vi "Autonomous Independent.vi"() -> ()   [LabVIEW 2017]
doc: "This VI is called when autonomous begins, and will automatically be terminated when autonomous ends. You can carry out timed or sensor driven robot movement independently without needing to return to the caller."
uses:
  Control 1.ctl
  Motion_Profiler_Class/Motion_Profiler_Class-323eb47bd4286328f3a3e236ed86bebf76c73fb1/MotionProfiles.lvclass
  <vilib>/Platform/TimedLoop/XDataNode/timing_clust.ctl
  <vilib>/Platform/TimedLoop/XDataNode/nitl_modes.ctl
  <vilib>/Platform/TimedLoop/XDataNode/wakeup.ctl
  <vilib>/Rock Robotics/WPI/Utilities/WPI_GetSetVariantRefNum.vi
  <vilib>/Rock Robotics/Network Tables/NT Write Numeric Array.vi
  <vilib>/Rock Robotics/Network Tables/NT Read String.vi
  UpperSwitchPressed.vi
  <vilib>/Platform/TimedLoop/XDataNode/XDataNode.xnode
  <vilib>/Platform/TimedLoop/XDataNode/XDNodeRunTimeDep.lvlib
panel:
  out "timer 2":u32=2247064
  out "AutoMode":string="LeftSwitch"
  out "MP Is Done Left":bool
  out "MP Is Done Right":bool
  in  "P_Right":dbl=0.25
  in  "I_Right":dbl
  in  "D_Right":dbl
  in  "F_Right":dbl=0.12
  in  "F_Left":dbl=0.12
  in  "D_Left":dbl
  in  "I_Left":dbl
  in  "P_Left":T1=0.19
  out "Right Bottom Buf Count":i32=5
  out "Right Is Under Run":bool
  out "Left Bottom Buf Count":i32=4
  out "Left Is Under Run":bool
  out "Left Vel":T2(graph)={"Set_Vel_(u/100ms)"=-8588, "Act_Vel_(u/100ms)"=-7311}
  out "Numeric":i32=26
  out "Right Vel":T2(graph)={"Set_Vel_(u/100ms)"=-8603, "Act_Vel_(u/100ms)"=-7623}
  out "Right Pos":T2(graph)={"Set_Vel_(u/100ms)"=-90788, "Act_Vel_(u/100ms)"=-97839}
  out "Left Pos":T2(graph)={"Set_Vel_(u/100ms)"=-72192, "Act_Vel_(u/100ms)"=-77390}
  out "Right Throttle":dbl(graph)=-0.9902248289345064
  out "Left Throttle":dbl(graph)=0.13880742913000976
  # "Be sure to right-click and choose Data Operations>>Make Current Value default if you want to save the array values with the VI"
  # "Left P gain: 0.21, Right P Gain 0.25 -> before 09/12/18\nLeft Gain :0.205, Right Gain .25 - > 09/12/18 -> Tuned after changing center drop for center grove practice"
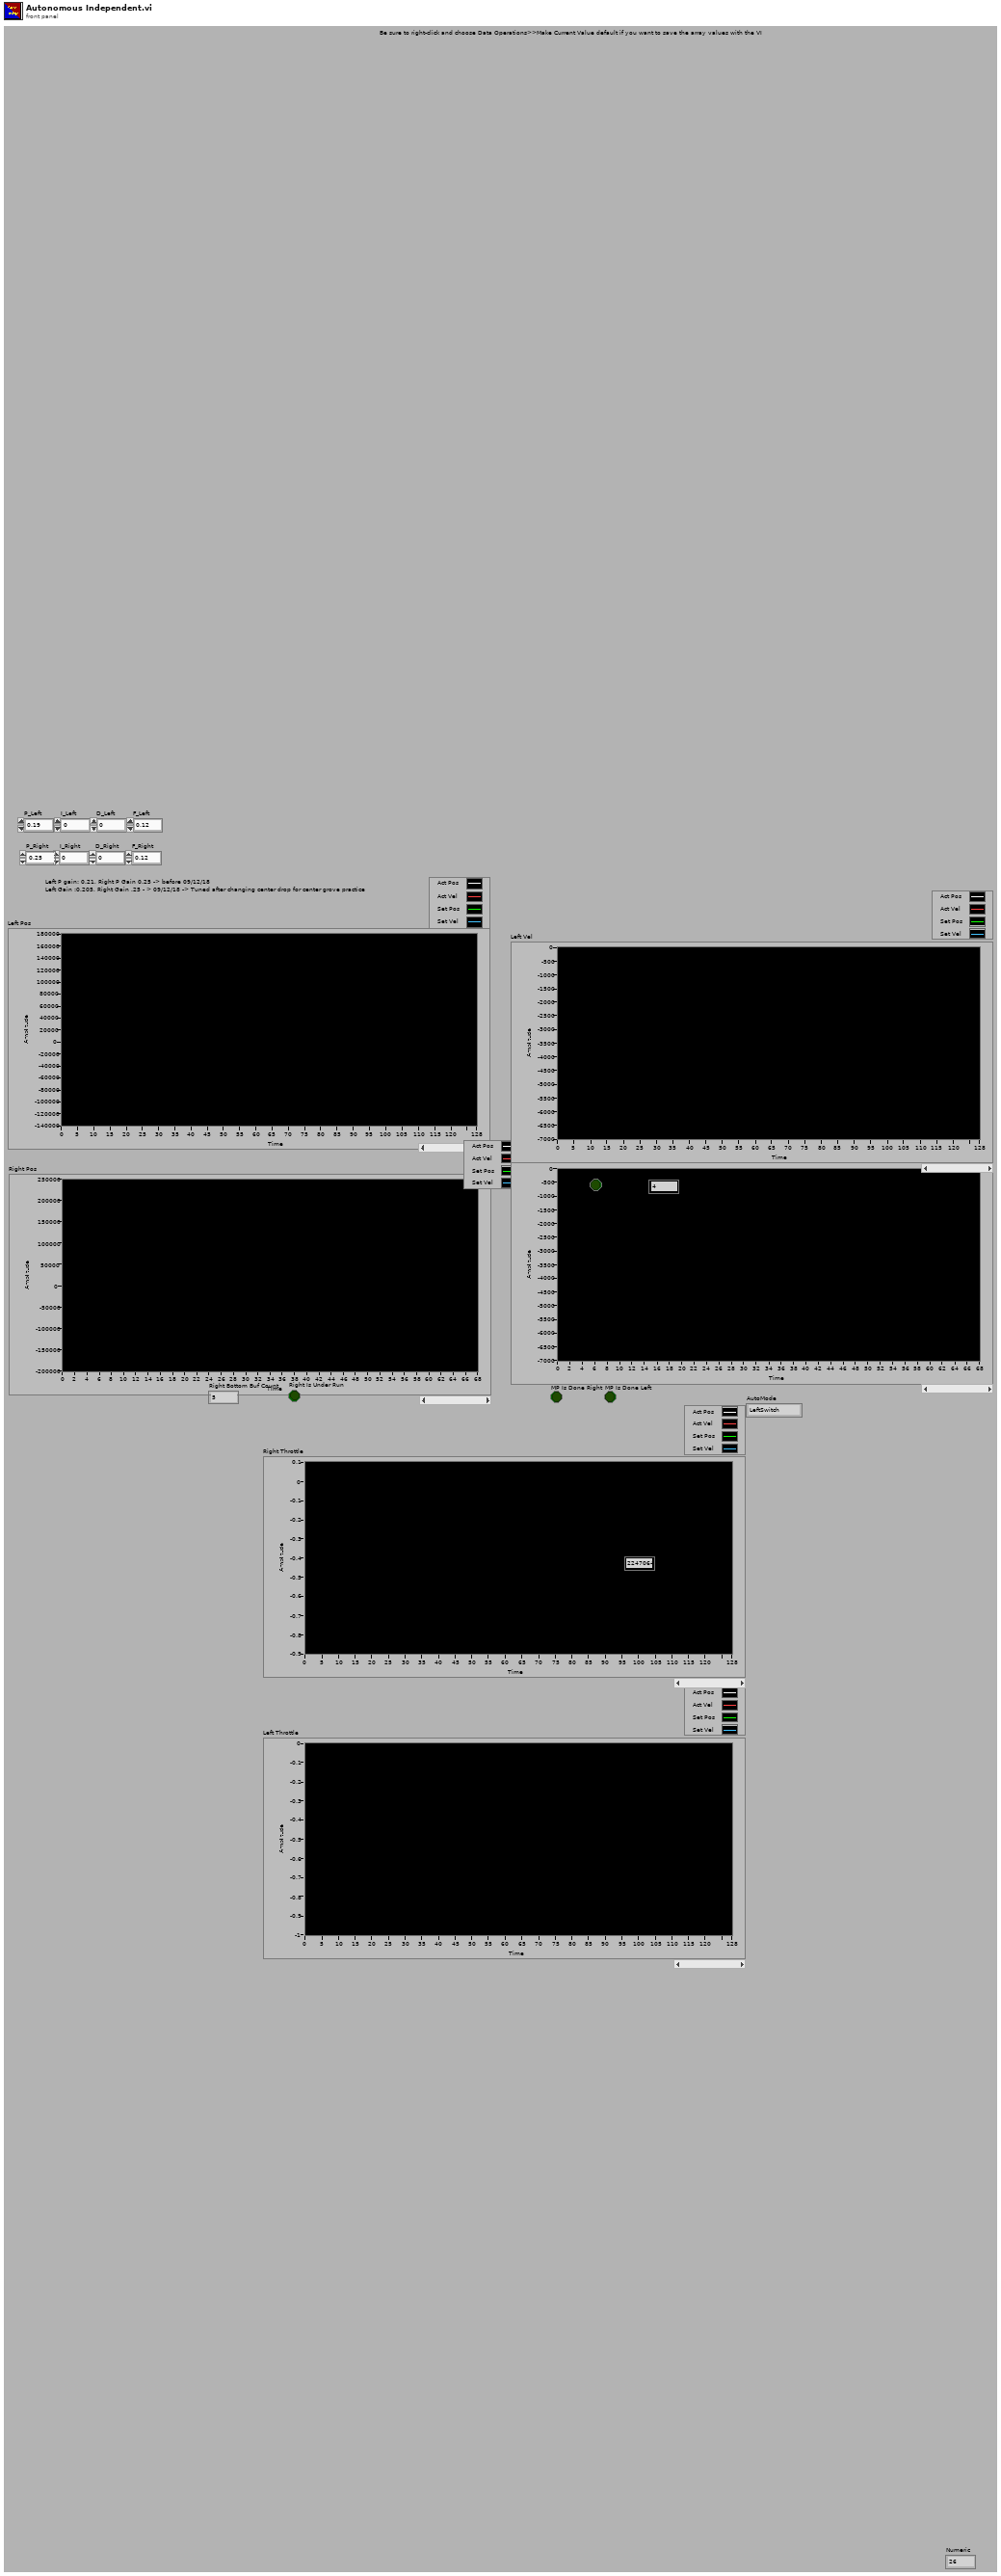
[diagram p1: front panel]
types:
  T1 = typedef "Control 1.ctl" = dbl
  T2 = cluster{"Set_Vel_(u/100ms)":i32, "Act_Vel_(u/100ms)":i32}
  T3 = typedef "WPI_JoystickDevRef.ctl" = cluster{"Device":T4}
  T4 = typedef "WPI_JoystickDeviceEnum.ctl" = enum16{"USB 0", "USB 1", "USB 2", "USB 3", "USB 4", "USB 5"}
  T5 = typedef "WPI_MotorControlDeviceRef.ctl" = cluster{"DeviceStatus":errorcluster, "Type":T6, "PWM":cluster{"PWM Channel":T7, "DeadBand":T8}, "CAN":cluster{"Device Number":u8, "SetOutput VI Ref":variant, "GetOutput VI Ref":variant, "Enable VI Ref":variant, "Disable VI Ref":variant, "Data":variant}, "Invert":bool, "DIO PWM":cluster{"PWM \"Enable\" Channel":T7, "DIOChannel":T9, "PWM Rate":dbl}}
  T6 = typedef "WPI_MotorControlType.ctl" = enum16{"PWM", "CAN", "DIO PWM"}
  T7 = typedef "FPGA_DIOPWMChannel.ctl" = enum8{"PWM 0", "PWM 1", "PWM 2", "PWM 3", "PWM 4", "PWM 5", "PWM 6", "PWM 7", "PWM 8", "PWM 9", "PWM MXP 0", "PWM MXP 1", "PWM MXP 2", "PWM MXP 3", "PWM MXP 4", "PWM MXP 5", "PWM MXP 6", "PWM MXP 7", "PWM MXP 8", "PWM MXP 9", "Invalid"}
  T8 = typedef "WPI_PWMDeadband.ctl" = cluster{"Name":string, "maxPositivePwm":i32, "minPositivePwm":i32, "centerPwm":i32, "maxNegativePwm":i32, "minNegativePwm":i32, "angularRange":u16}
  T9 = typedef "FPGA_DIOChannel.ctl" = enum8{"DIO 0", "DIO 1", "DIO 2", "DIO 3", "DIO 4", "DIO 5", "DIO 6", "DIO 7", "DIO 8", "DIO 9", "DIO MXP 0", "DIO MXP 1", "DIO MXP 2", "DIO MXP 3", "DIO MXP 4", "DIO MXP 5", "DIO MXP 6", "DIO MXP 7", "DIO MXP 8", "DIO MXP 9", "DIO MXP 10", "DIO MXP 11", "DIO MXP 12", "DIO MXP 13", "DIO MXP 14", "DIO MXP 15", "SPI Port CS1", "SPI Port CS2", "SPI Port CS3", "SPI Port MISO", "SPI Port MOSI", "Invalid"}
  T10 = typedef "XDNodeRunTimeDep.lvlib/timing_clust.ctl" = cluster{"Expected End [f-1]":u64, "Actual End [f-1]":u64, "Finished Late? [f-1]":bool, "Expected End [i-1]":u64, "Actual End [i-1]":u64, "Finished Late? [i-1]":bool, "Expected Start [i]":u64, "Actual Start [i]":u64, "Expected Start [f]":u64, "Actual Start [f]":u64, "Source Name":string, "Structure Name":string, "Period":i64, "Deadline":i64, "Offset":i64, "Start":i64, "Priority":i32, "Timeout":i32, "Mode":T11, "Wakeup Reason":T12, "Error":errorcluster, "Source Type":string, "Secondary Source Type":string, "Global End Time":u64, "Global Start Time":u64, "Frame Duration":u64, "Iteration Duration":u64, "Assigned CPU":i32, "I/O Scan Engine Mode":u32}
  T11 = typedef "XDNodeRunTimeDep.lvlib/nitl_modes.ctl" = enum32{"No Change", "Process missed periods, maintain original phase", "Discard missed periods, maintain original phase", "Process missed periods, ignore original phase", "Discard missed periods, ignore original phase"}
  T12 = typedef "XDNodeRunTimeDep.lvlib/wakeup.ctl" = enum32{"Normal", "Aborted", "Asynchronous wakeup", "Timing source error", "Timed loop error", "Timeout"}
  T13 = typedef "MotionProfiles.lvclass/MotionProfile_MP_Class_Status.ctl" = cluster{"Motion Profile Status":cluster{"Top Buffer Remaining":i32, "Top Buffer Count":i32, "Bottom Buffer Count":i32, "Has Underrun?":bool, "Is Underrun?":bool, "Active Point Valid?":bool, "Is Last?":bool, "Profile Slot Select 0":i32, "Output Enable":i32, "Time Duration (ms)":i32, "Profile Slot Select 1":i32}, "TalonState":T14, "MP Is Done":bool, "MP Is Executing":bool, "Set_Vel_(u/100ms)":i32, "Set_Pos_(u)":i32, "Act_Vel_(u/100ms)":i32, "Act_Pos(u)":i32, "Throtle":dbl}
  T14 = typedef "MotionProfiles.lvclass/MotionProfile_TalonSetValueEnum.ctl" = enum16{"Disable", "Enable", "Hold"}
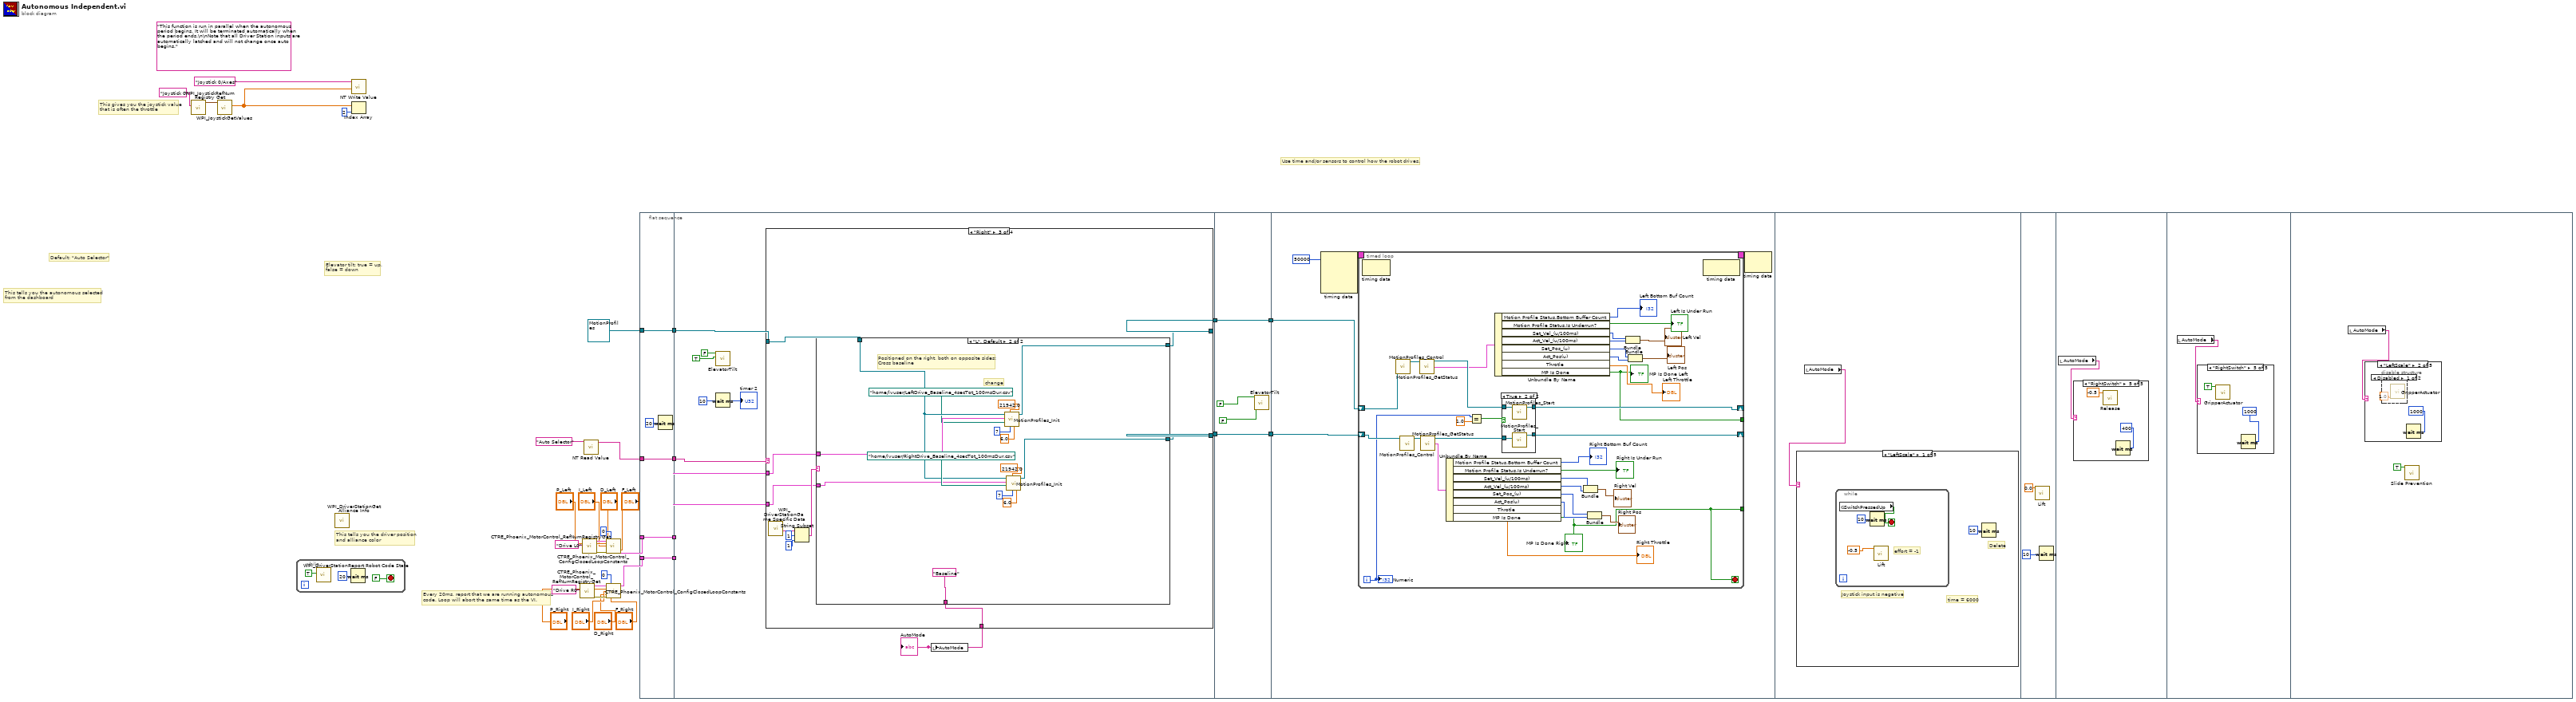
[diagram p0: block diagram]
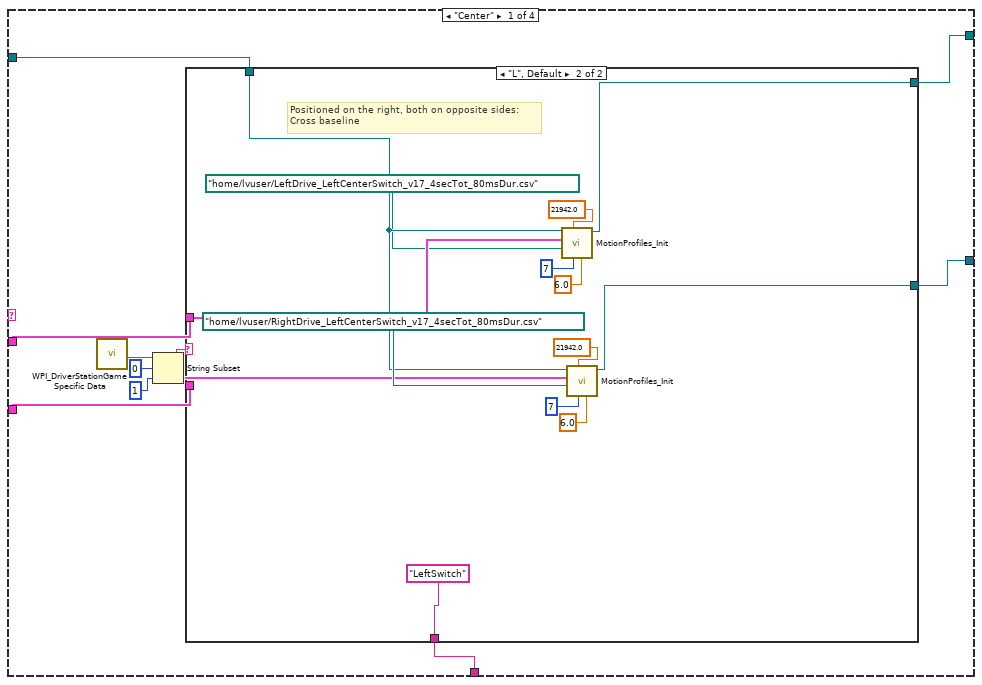
[diagram p2: hidden frame]
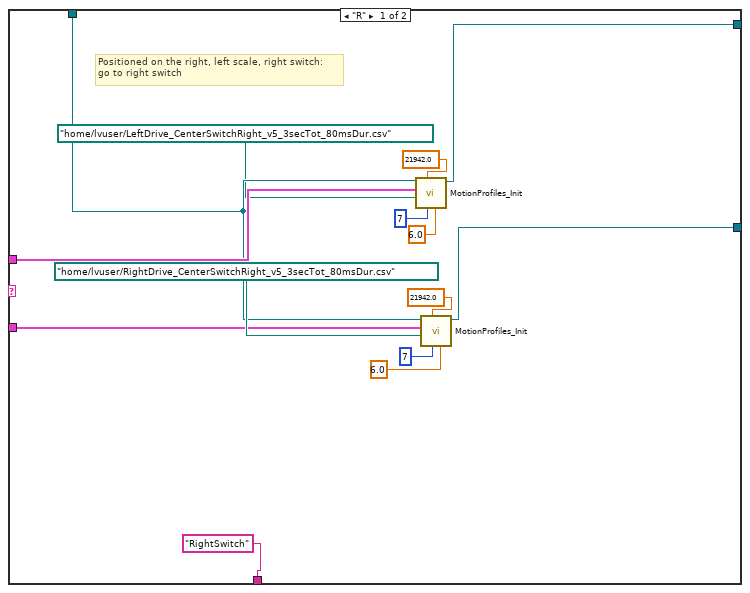
[diagram p3: hidden frame]
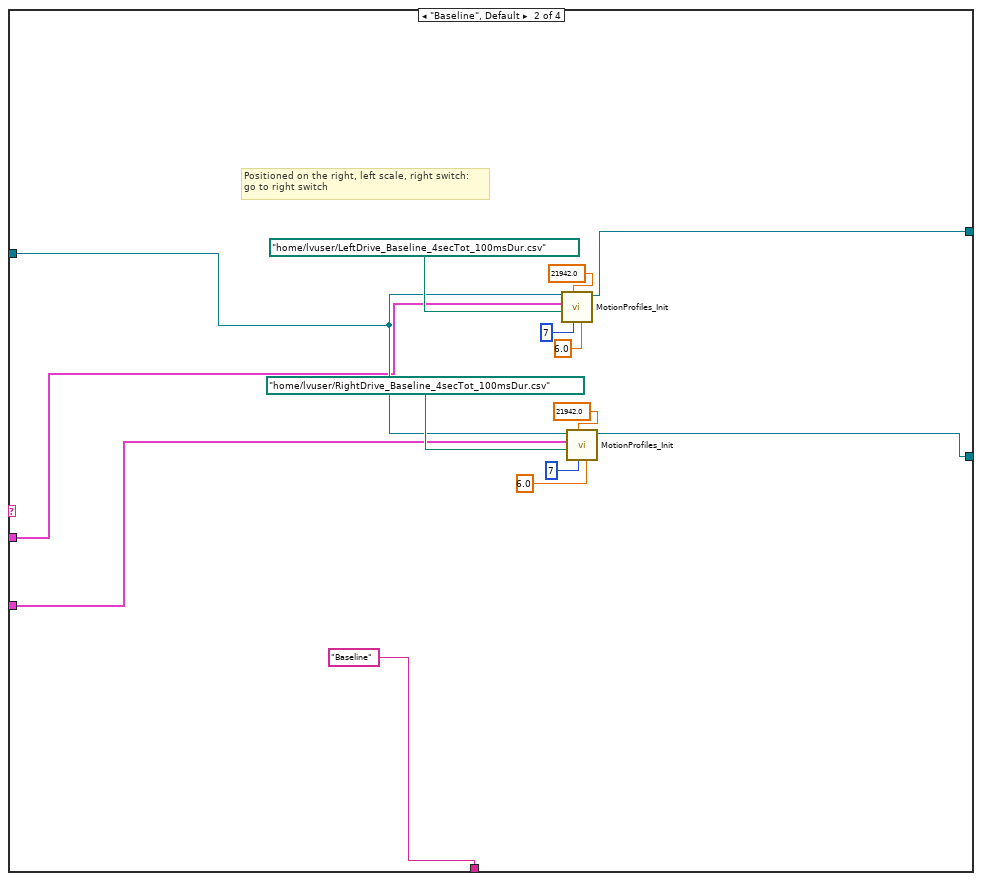
[diagram p4: hidden frame]
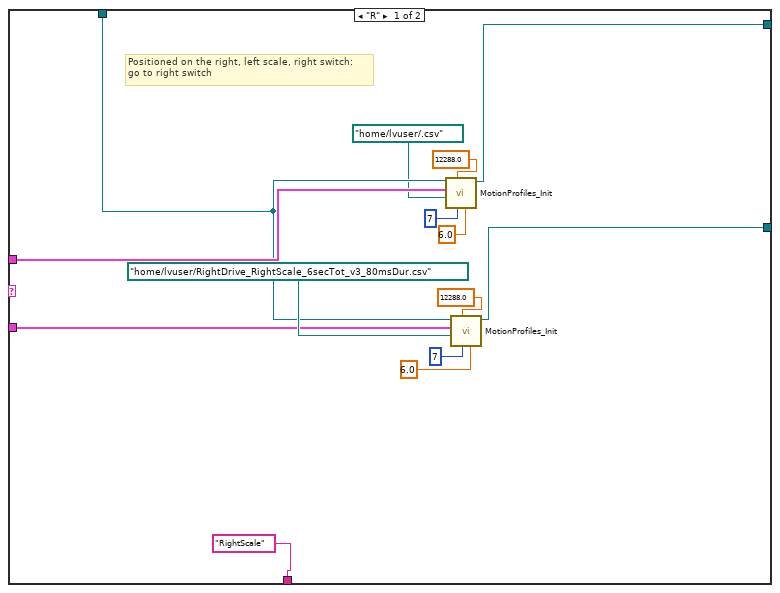
[diagram p5: hidden frame]
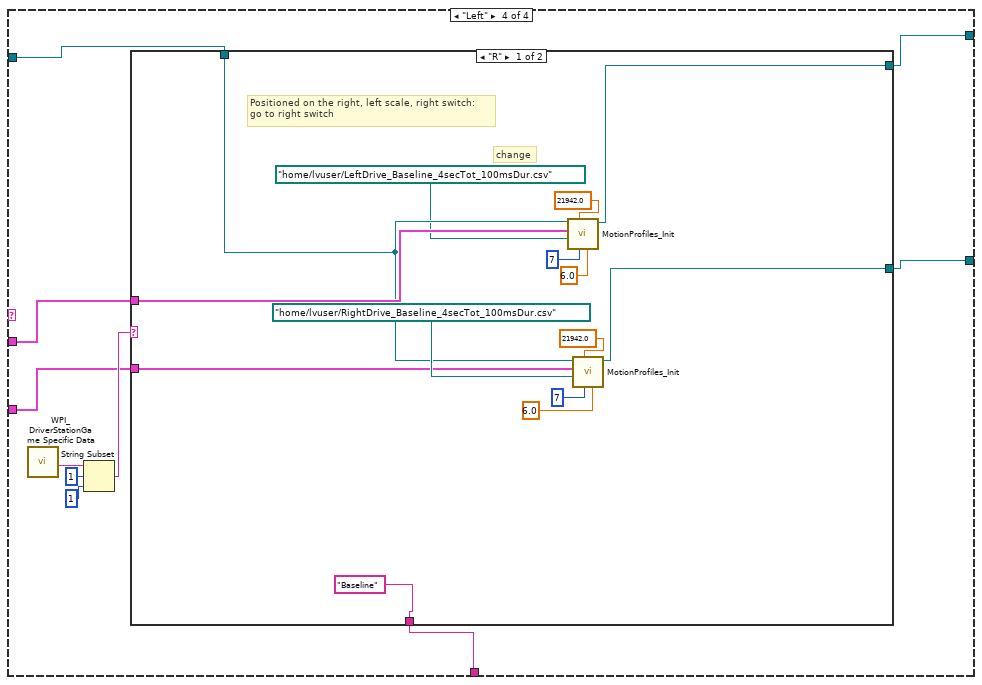
[diagram p6: hidden frame]
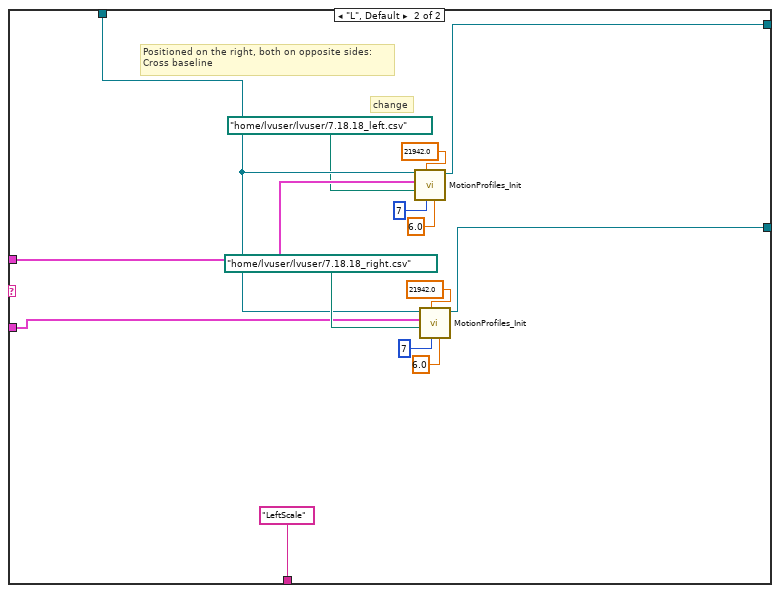
[diagram p7: hidden frame]
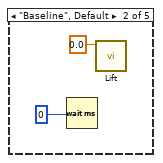
[diagram p9: hidden frame]
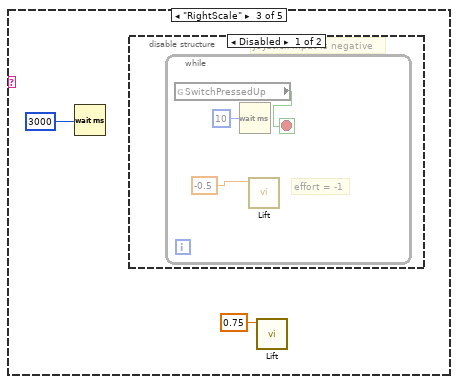
[diagram p10: hidden frame]
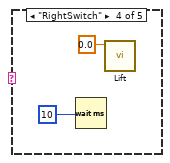
[diagram p12: hidden frame]
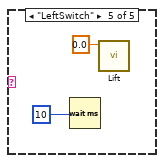
[diagram p13: hidden frame]
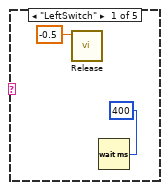
[diagram p14: hidden frame]
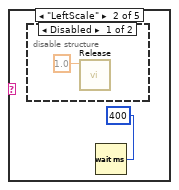
[diagram p15: hidden frame]
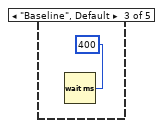
[diagram p17: hidden frame]
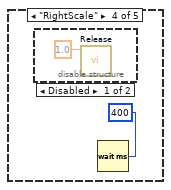
[diagram p18: hidden frame]
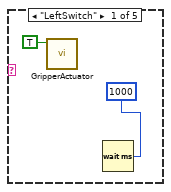
[diagram p20: hidden frame]
diagram:
  (unwired) "This function is run in parallel when the autonomous period begins. It will be terminated automatically when the period ends.\n\nNote that all Driver Station inputs are automatically latched and will not change once auto begins."
  # "Elevator tilt: true = up,\nfalse = down"
  # "Every 20ms, report that we are running autonomous\ncode. Loop will abort the same time as the VI."
  # "Default: \"Auto Selector\""
  # "This tells you the autonomous selected\nfrom the dashboard"
  # "This gives you the joystick value\nthat is often the throttle"
  # "Use time and/or sensors to control how the robot drives."
  # "This tells you the driver position\nand alliance color"
  n1 = call <vilib>:"WPI_JoystickRefNum Registry Get.vi"("refnum name"="Joystick 0") -> ("JoystickDevRef"=w33:T3)  [unwired: 1 in, 9 out]
  n2 = call <vilib>:"WPI_JoystickGetValues.vi"("JoystickDevRef"=w33) -> ("Axes"=w31:dbl[])  [unwired: 6 in, 4 out]
  n3 = while {
    stop <- FALSE stop-if-true
    n4 = call <vilib>:"WPI_DriverStationReport Robot Code State.vi"("Autonomous"=TRUE) -> ()  [unwired: 10 in, 1 out]
    n5 = Wait (ms)(milliseconds to wait=u32 20) -> ()  [unwired: 1 out]
  }
  n6 = call <vilib>:"WPI_DriverStationGet Alliance Info.vi"() -> ()  [unwired: 12 out]
  n7 = call-poly <vilib>:"NT Write Value.vi"("Numeric Array"=w31, "Name"="Joystick 0/Axes") -> ()  [unwired: 9 in, 1 out]
  n8 = Index Array(array=w31, index=2) -> ()  [unwired: 1 out]
  n9 = call <vilib>:"CTRE_Phoenix_MotorControl_RefNumRegistryGet.vi"("refnum name"="Drive R0") -> ("error out"=w21:errorcluster, "PhoenixMotorControlDevRef"=w22:T5)  [unwired: 9 in]
  n10 = call <vilib>:"CTRE_Phoenix_MotorControl_RefNumRegistryGet.vi"("refnum name"="Drive L0") -> ("error out"=w24:errorcluster, "PhoenixMotorControlDevRef"=w25:T5)  [unwired: 9 in]
  n11 = call-poly <vilib>:"NT Read Value.vi"("Name"="Auto Selector") -> ("String"=w5:string)  [unwired: 9 in, 1 out]
  n12 = call <vilib>:"CTRE_Phoenix_MotorControl_ConfigClosedLoopConstants.vi"("PhoenixMotorControlDevRef"=w25, "slotIdx"=0, "P"="P_Left", "I"="I_Left", "D"="D_Left", "error in (no error)"=w24, "F"="F_Left") -> ("PhoenixMotorControlDevRef"=w18:T5)  [unwired: 7 in, 1 out]
  n13 = call <vilib>:"CTRE_Phoenix_MotorControl_ConfigClosedLoopConstants.vi"("PhoenixMotorControlDevRef"=w22, "slotIdx"=0, "P"="P_Right", "I"="I_Right", "D"="D_Right", "error in (no error)"=w21, "F"="F_Right") -> ("PhoenixMotorControlDevRef"=w17:T5)  [unwired: 7 in, 1 out]
  n14 = flat-sequence {
    tunnel: w5 -> [w39]
    tunnel: refnum<class "MotionProfiles.lvclass"> refnum ("MotionProfiles.lvclass") -> [w40]
    tunnel: w17 -> [w41]
    tunnel: w18 -> [w42]
    tunnel: [w42] -> w10
    tunnel: [w41] -> w9
    tunnel: [w40] -> w8
    tunnel: [w39] -> w7
    tunnel: [w50] -> w2
    tunnel: [w51] -> w1
    tunnel: w10 -> [w53]
    tunnel: w9 -> [w52]
    tunnel: w8 -> [w49]
    tunnel: w7 -> [w47]
    tunnel: w2 -> [w185]
    tunnel: [w185] -> w4
    tunnel: w1 -> [w184]
    tunnel: [w184] -> w3
    tunnel: w4 -> [w190]
    tunnel: w3 -> [w189]
    frame #0 {
      n15 = Wait (ms)(milliseconds to wait=u32 20) -> ()  [unwired: 1 out]
    }
    frame #1 {
      n16 = call "ElevatorTilt.vi"("Down?"=TRUE, "Up"=FALSE) -> ()  [unwired: 10 in]
      n17 = Wait (ms)(milliseconds to wait=u32 10) -> (millisecond timer value=→"timer 2":u32)
      n18 = case shown="\"Right\"" w47 {
        tunnel: w53 -> [w62 w94 w110 w148]
        tunnel: w52 -> [w61 w93 w109 w147]
        tunnel: [w60 w95 w106 w144] -> w51
        tunnel: [w59 w96 w107 w145] -> w50
        tunnel: w49 -> [w55 w97 w115 w149]
        tunnel: [w54 "Baseline" w108 w146] -> w48
        frame "Center" {
          n19 = call <vilib>:"WPI_DriverStationGame Specific Data.vi"() -> ("Game Specific Data"=w63:string)  [unwired: 11 in]
          n20 = String Subset(string=w63, offset (0)=0, length (rest)=1 ("length (rest)")) -> (substring=w58:string)
          n21 = case shown="\"L\", Default" w58 {
            tunnel: w62 -> [w70 w83]
            tunnel: w61 -> [w69 w84]
            tunnel: [w68 w82] -> w59
            tunnel: [w67 w81] -> w60
            tunnel: w55 -> [w66 w80]
            tunnel: ["RightSwitch" "LeftSwitch"] -> w54
            frame "R" {
              # "Positioned on the right, left scale, right switch:\ngo to right switch"
              n22 = call "MotionProfiles_Init.vi"("Wheel_Diameter (in)"=6.0, "MP_Frame_Rate_(ms)"=7, "Encoder_CPR_4x"=21942.0, "CSV File Path"=path "/home/lvuser/LeftDrive_CenterSwitchRight_v5_3secTot_80msDur.csv", "PhoenixMotorControlDevRef"=w70, "MotionProfiles in"=w66) -> ("MotionProfiles out"=w68:refnum<class "MotionProfiles.lvclass">)  [unwired: 4 in, 1 out]
              n23 = call "MotionProfiles_Init.vi"("Wheel_Diameter (in)"=6.0, "MP_Frame_Rate_(ms)"=7, "Encoder_CPR_4x"=21942.0, "CSV File Path"=path "/home/lvuser/RightDrive_CenterSwitchRight_v5_3secTot_80msDur.csv", "PhoenixMotorControlDevRef"=w69, "MotionProfiles in"=w66) -> ("MotionProfiles out"=w67:refnum<class "MotionProfiles.lvclass">)  [unwired: 4 in, 1 out]
            }
            frame "L", Default {
              # "Positioned on the right, both on opposite sides:\nCross baseline"
              n24 = call "MotionProfiles_Init.vi"("Wheel_Diameter (in)"=6.0, "MP_Frame_Rate_(ms)"=7, "Encoder_CPR_4x"=21942.0, "CSV File Path"=path "/home/lvuser/LeftDrive_LeftCenterSwitch_v17_4secTot_80msDur.csv", "PhoenixMotorControlDevRef"=w83, "MotionProfiles in"=w80) -> ("MotionProfiles out"=w82:refnum<class "MotionProfiles.lvclass">)  [unwired: 4 in, 1 out]
              n25 = call "MotionProfiles_Init.vi"("Wheel_Diameter (in)"=6.0, "MP_Frame_Rate_(ms)"=7, "Encoder_CPR_4x"=21942.0, "CSV File Path"=path "/home/lvuser/RightDrive_LeftCenterSwitch_v17_4secTot_80msDur.csv", "PhoenixMotorControlDevRef"=w84, "MotionProfiles in"=w80) -> ("MotionProfiles out"=w81:refnum<class "MotionProfiles.lvclass">)  [unwired: 4 in, 1 out]
            }
          }
        }
        frame "Baseline", Default {
          # "Positioned on the right, left scale, right switch:\ngo to right switch"
          n26 = call "MotionProfiles_Init.vi"("Wheel_Diameter (in)"=6.0, "MP_Frame_Rate_(ms)"=7, "Encoder_CPR_4x"=21942.0, "CSV File Path"=path "/home/lvuser/LeftDrive_Baseline_4secTot_100msDur.csv", "PhoenixMotorControlDevRef"=w94, "MotionProfiles in"=w97) -> ("MotionProfiles out"=w96:refnum<class "MotionProfiles.lvclass">)  [unwired: 4 in, 1 out]
          n27 = call "MotionProfiles_Init.vi"("Wheel_Diameter (in)"=6.0, "MP_Frame_Rate_(ms)"=7, "Encoder_CPR_4x"=21942.0, "CSV File Path"=path "/home/lvuser/RightDrive_Baseline_4secTot_100msDur.csv", "PhoenixMotorControlDevRef"=w93, "MotionProfiles in"=w97) -> ("MotionProfiles out"=w95:refnum<class "MotionProfiles.lvclass">)  [unwired: 4 in, 1 out]
        }
        frame "Right" {
          n28 = call <vilib>:"WPI_DriverStationGame Specific Data.vi"() -> ("Game Specific Data"=w114:string)  [unwired: 11 in]
          n29 = String Subset(string=w114, offset (0)=1, length (rest)=1 ("length (rest)")) -> (substring=w111:string)
          n30 = case shown="\"L\", Default" w111 {
            tunnel: w110 -> [w122 w135]
            tunnel: w109 -> [w121 w136]
            tunnel: [w120 w134] -> w107
            tunnel: [w119 w133] -> w106
            tunnel: w115 -> [w118 w132]
            tunnel: ["RightScale" "Baseline"] -> w108
            frame "R" {
              # "Positioned on the right, left scale, right switch:\ngo to right switch"
              n31 = call "MotionProfiles_Init.vi"("Wheel_Diameter (in)"=6.0, "MP_Frame_Rate_(ms)"=7, "Encoder_CPR_4x"=12288.0, "CSV File Path"=path "/home/lvuser/.csv", "PhoenixMotorControlDevRef"=w122, "MotionProfiles in"=w118) -> ("MotionProfiles out"=w120:refnum<class "MotionProfiles.lvclass">)  [unwired: 4 in, 1 out]
              n32 = call "MotionProfiles_Init.vi"("Wheel_Diameter (in)"=6.0, "MP_Frame_Rate_(ms)"=7, "Encoder_CPR_4x"=12288.0, "CSV File Path"=path "/home/lvuser/RightDrive_RightScale_6secTot_v3_80msDur.csv", "PhoenixMotorControlDevRef"=w121, "MotionProfiles in"=w118) -> ("MotionProfiles out"=w119:refnum<class "MotionProfiles.lvclass">)  [unwired: 4 in, 1 out]
            }
            frame "L", Default {
              # "change"
              # "Positioned on the right, both on opposite sides:\nCross baseline"
              n33 = call "MotionProfiles_Init.vi"("Wheel_Diameter (in)"=6.0, "MP_Frame_Rate_(ms)"=7, "Encoder_CPR_4x"=21942.0, "CSV File Path"=path "/home/lvuser/LeftDrive_Baseline_4secTot_100msDur.csv", "PhoenixMotorControlDevRef"=w135, "MotionProfiles in"=w132) -> ("MotionProfiles out"=w134:refnum<class "MotionProfiles.lvclass">)  [unwired: 4 in, 1 out]
              n34 = call "MotionProfiles_Init.vi"("Wheel_Diameter (in)"=6.0, "MP_Frame_Rate_(ms)"=7, "Encoder_CPR_4x"=21942.0, "CSV File Path"=path "/home/lvuser/RightDrive_Baseline_4secTot_100msDur.csv", "PhoenixMotorControlDevRef"=w136, "MotionProfiles in"=w132) -> ("MotionProfiles out"=w133:refnum<class "MotionProfiles.lvclass">)  [unwired: 4 in, 1 out]
            }
          }
        }
        frame "Left" {
          n35 = call <vilib>:"WPI_DriverStationGame Specific Data.vi"() -> ("Game Specific Data"=w153:string)  [unwired: 11 in]
          n36 = String Subset(string=w153, offset (0)=1, length (rest)=1 ("length (rest)")) -> (substring=w150:string)
          n37 = case shown="\"R\"" w150 {
            tunnel: w148 -> [w160 w173]
            tunnel: w147 -> [w159 w174]
            tunnel: [w158 w172] -> w145
            tunnel: [w157 w171] -> w144
            tunnel: w149 -> [w156 w170]
            tunnel: ["Baseline" "LeftScale"] -> w146
            frame "R" {
              # "change"
              # "Positioned on the right, left scale, right switch:\ngo to right switch"
              n38 = call "MotionProfiles_Init.vi"("Wheel_Diameter (in)"=6.0, "MP_Frame_Rate_(ms)"=7, "Encoder_CPR_4x"=21942.0, "CSV File Path"=path "/home/lvuser/LeftDrive_Baseline_4secTot_100msDur.csv", "PhoenixMotorControlDevRef"=w160, "MotionProfiles in"=w156) -> ("MotionProfiles out"=w158:refnum<class "MotionProfiles.lvclass">)  [unwired: 4 in, 1 out]
              n39 = call "MotionProfiles_Init.vi"("Wheel_Diameter (in)"=6.0, "MP_Frame_Rate_(ms)"=7, "Encoder_CPR_4x"=21942.0, "CSV File Path"=path "/home/lvuser/RightDrive_Baseline_4secTot_100msDur.csv", "PhoenixMotorControlDevRef"=w159, "MotionProfiles in"=w156) -> ("MotionProfiles out"=w157:refnum<class "MotionProfiles.lvclass">)  [unwired: 4 in, 1 out]
            }
            frame "L", Default {
              # "change"
              # "Positioned on the right, both on opposite sides:\nCross baseline"
              n40 = call "MotionProfiles_Init.vi"("Wheel_Diameter (in)"=6.0, "MP_Frame_Rate_(ms)"=7, "Encoder_CPR_4x"=21942.0, "CSV File Path"=path "/home/lvuser/lvuser/7.18.18_left.csv", "PhoenixMotorControlDevRef"=w173, "MotionProfiles in"=w170) -> ("MotionProfiles out"=w172:refnum<class "MotionProfiles.lvclass">)  [unwired: 4 in, 1 out]
              n41 = call "MotionProfiles_Init.vi"("Wheel_Diameter (in)"=6.0, "MP_Frame_Rate_(ms)"=7, "Encoder_CPR_4x"=21942.0, "CSV File Path"=path "/home/lvuser/lvuser/7.18.18_right.csv", "PhoenixMotorControlDevRef"=w174, "MotionProfiles in"=w170) -> ("MotionProfiles out"=w171:refnum<class "MotionProfiles.lvclass">)  [unwired: 4 in, 1 out]
            }
          }
        }
      }
      "AutoMode" <- w48
      n42 = local write "AutoMode"(w48) -> ()
    }
    frame #2 {
      n43 = call "ElevatorTilt.vi"("Down?"=FALSE, "Up"=FALSE) -> ()  [unwired: 10 in]
    }
    frame #3 {
      n44 = node-c288(50000) -> (w188:T10)  [unwired: 3 in]
      n45 = timed-loop {
        timing: w188 -> [_]
        timing-out: [_] -> w187
        shift-right: [w211] -> _
        shift-left: w189 -> [w209]
        shift-right: [w210] -> _
        shift-left: w190 -> [w193]
        tunnel: [w191] -> _
        tunnel: [w192] -> _
        i -> [w206]
        stop <- w191 stop-if-true
        n46 = node-c288() -> ()  [unwired: 1 in, 1 out]
        n47 = call "MotionProfiles_Control.vi"("MotionProfiles in"=w193) -> ("MotionProfiles out"=w223:refnum<class "MotionProfiles.lvclass">)  [unwired: 9 in, 1 out]
        n48 = call "MotionProfiles_Control.vi"("MotionProfiles in"=w209) -> ("MotionProfiles out"=w222:refnum<class "MotionProfiles.lvclass">)  [unwired: 9 in, 1 out]
        n49 = call "MotionProfiles_GetStatus.vi"("MotionProfiles in"=w223) -> ("MotionProfiles out"=w220:refnum<class "MotionProfiles.lvclass">, "MP_Class_Status"=w218:T13)  [unwired: 12 in, 1 out]
        n50 = call "MotionProfiles_GetStatus.vi"("MotionProfiles in"=w222) -> ("MotionProfiles out"=w221:refnum<class "MotionProfiles.lvclass">, "MP_Class_Status"=w219:T13)  [unwired: 12 in, 1 out]
        n51 = Unbundle By Name(w219) -> ("Motion Profile Status.Bottom Buffer Count"=→"Right Bottom Buf Count":i32, "Motion Profile Status.Is Underrun?"=→"Right Is Under Run":bool, "Set_Vel_(u/100ms)"=w203:i32, "Act_Vel_(u/100ms)"=w202:i32, "Set_Pos_(u)"=w200:i32, "Act_Pos(u)"=w199:i32, "Throtle"=→"Right Throttle":dbl, "MP Is Done"=w191:bool)
        "MP Is Done Right" <- w191
        n52 = Equal?(x=w206, y=1.0) -> (x = y?=w208:bool)
        n53 = Unbundle By Name(w218) -> ("Motion Profile Status.Bottom Buffer Count"=→"Left Bottom Buf Count":i32, "Motion Profile Status.Is Underrun?"=→"Left Is Under Run":bool, "Set_Vel_(u/100ms)"=w205:i32, "Act_Vel_(u/100ms)"=w213:i32, "Set_Pos_(u)"=w197:i32, "Act_Pos(u)"=w196:i32, "Throtle"=→"Left Throttle":dbl, "MP Is Done"=w192:bool)
        "MP Is Done Left" <- w192
        n54 = case shown="True" w208 {
          tunnel: w221 -> [w224 w229]
          tunnel: w220 -> [w225 w228]
          tunnel: [w224 w227] -> w211
          tunnel: [w225 w226] -> w210
          frame False {
          }
          frame True {
            n55 = call "MotionProfiles_Start.vi"("MotionProfiles in"=w228) -> ("MotionProfiles out"=w226:refnum<class "MotionProfiles.lvclass">)  [unwired: 9 in, 1 out]
            n56 = call "MotionProfiles_Start.vi"("MotionProfiles in"=w229) -> ("MotionProfiles out"=w227:refnum<class "MotionProfiles.lvclass">)  [unwired: 9 in, 1 out]
          }
        }
        n57 = Bundle("Set_Vel_(u/100ms)"=w203, "Act_Vel_(u/100ms)"=w202) -> (→"Right Vel":T2)  [unwired: 1 in]
        n58 = Bundle("Set_Pos_(u)"=w200, "Act_Pos(u)"=w199) -> (→"Right Pos":cluster{"Set_Pos_(u)":i32, "Act_Pos(u)":i32})  [unwired: 1 in]
        n59 = Bundle("Set_Vel_(u/100ms)"=w205, "Act_Vel_(u/100ms)"=w213) -> (→"Left Vel":T2)  [unwired: 1 in]
        n60 = Bundle("Set_Pos_(u)"=w197, "Act_Pos(u)"=w196) -> (→"Left Pos":cluster{"Set_Pos_(u)":i32, "Act_Pos(u)":i32})  [unwired: 1 in]
        n61 = node-c288() -> ()  [unwired: 1 in, 1 out]
        "Numeric" <- w206
      }
      n62 = node-c288(w187) -> ()  [unwired: 1 out]
    }
    frame #4 {
      n63 = local read "AutoMode"() -> (w236:string)
      n64 = case shown="\"LeftScale\"" w236 {
        frame "LeftScale" {
          # "Delete"
          # "time = 6000"
          # "Joystick input is negative"
          n65 = while {
            stop <- w240 stop-if-true
            # "effort = -1"
            n66 = global read "UpperSwitchPressed.vi" "SwitchPressedUp"() -> (w240:bool)
            n67 = Wait (ms)(milliseconds to wait=u32 10) -> ()  [unwired: 1 out]
            n68 = call "Lift.vi"("Effort"=-0.5) -> ()  [unwired: 11 in]
          }
          n69 = Wait (ms)(milliseconds to wait=u32 10) -> ()  [unwired: 1 out]
        }
        frame "Baseline", Default {
          n70 = Wait (ms)(milliseconds to wait=u32 0) -> ()  [unwired: 1 out]
          n71 = call "Lift.vi"("Effort"=0.0) -> ()  [unwired: 11 in]
        }
        frame "RightScale" {
          # "Joystick input is negative"
          n72 = Wait (ms)(milliseconds to wait=u32 3000) -> ()  [unwired: 1 out]
          n73 = disable-structure shown="Disabled" {
            frame Disabled {
              n74 = while {
                stop <- w247 stop-if-true
                # "effort = -1"
                n75 = global read "UpperSwitchPressed.vi" "SwitchPressedUp"() -> (w247:bool)
                n76 = Wait (ms)(milliseconds to wait=u32 10) -> ()  [unwired: 1 out]
                n77 = call "Lift.vi"("Effort"=-0.5) -> ()  [unwired: 11 in]
              }
            }
            frame Enabled {
            }
          }
          n78 = call "Lift.vi"("Effort"=0.75) -> ()  [unwired: 11 in]
        }
        frame "RightSwitch" {
          n79 = Wait (ms)(milliseconds to wait=u32 10) -> ()  [unwired: 1 out]
          n80 = call "Lift.vi"("Effort"=0.0) -> ()  [unwired: 11 in]
        }
        frame "LeftSwitch" {
          n81 = Wait (ms)(milliseconds to wait=u32 10) -> ()  [unwired: 1 out]
          n82 = call "Lift.vi"("Effort"=0.0) -> ()  [unwired: 11 in]
        }
      }
    }
    frame #5 {
      n83 = call "Lift.vi"("Effort"=0.0) -> ()  [unwired: 11 in]
      n84 = Wait (ms)(milliseconds to wait=u32 10) -> ()  [unwired: 1 out]
    }
    frame #6 {
      n85 = local read "AutoMode"() -> (w254:string)
      n86 = case shown="\"RightSwitch\"" w254 {
        frame "LeftSwitch" {
          n87 = call "Release.vi"("Release"=-0.5) -> ()  [unwired: 11 in]
          n88 = Wait (ms)(milliseconds to wait=u32 400) -> ()  [unwired: 1 out]
        }
        frame "LeftScale" {
          n89 = disable-structure shown="Disabled" {
            frame Disabled {
              n90 = call "Release.vi"("Release"=1.0) -> ()  [unwired: 11 in]
            }
            frame Enabled {
            }
          }
          n91 = Wait (ms)(milliseconds to wait=u32 400) -> ()  [unwired: 1 out]
        }
        frame "Baseline", Default {
          n92 = Wait (ms)(milliseconds to wait=u32 400) -> ()  [unwired: 1 out]
        }
        frame "RightScale" {
          n93 = disable-structure shown="Disabled" {
            frame Disabled {
              n94 = call "Release.vi"("Release"=1.0) -> ()  [unwired: 11 in]
            }
            frame Enabled {
            }
          }
          n95 = Wait (ms)(milliseconds to wait=u32 400) -> ()  [unwired: 1 out]
        }
        frame "RightSwitch" {
          n96 = call "Release.vi"("Release"=-0.5) -> ()  [unwired: 11 in]
          n97 = Wait (ms)(milliseconds to wait=u32 400) -> ()  [unwired: 1 out]
        }
      }
    }
    frame #7 {
      n98 = local read "AutoMode"() -> (w264:string)
      n99 = case shown="\"RightSwitch\"" w264 {
        frame "LeftSwitch" {
          n100 = call "GripperActuator.vi"("Up"=TRUE) -> ()  [unwired: 11 in]
          n101 = Wait (ms)(milliseconds to wait=u32 1000) -> ()  [unwired: 1 out]
        }
        frame "LeftScale" {
          n102 = disable-structure shown="Disabled" {
            frame Disabled {
              n103 = call "GripperActuator.vi"("Up"=TRUE) -> ()  [unwired: 11 in]
            }
            frame Enabled {
            }
          }
          n104 = Wait (ms)(milliseconds to wait=u32 1000) -> ()  [unwired: 1 out]
        }
        frame "Baseline", Default {
          n105 = Wait (ms)(milliseconds to wait=u32 1000) -> ()  [unwired: 1 out]
        }
        frame "RightScale" {
          n106 = disable-structure shown="Disabled" {
            frame Disabled {
              n107 = call "GripperActuator.vi"("Up"=TRUE) -> ()  [unwired: 11 in]
            }
            frame Enabled {
            }
          }
          n108 = Wait (ms)(milliseconds to wait=u32 1000) -> ()  [unwired: 1 out]
        }
        frame "RightSwitch" {
          n109 = call "GripperActuator.vi"("Up"=TRUE) -> ()  [unwired: 11 in]
          n110 = Wait (ms)(milliseconds to wait=u32 1000) -> ()  [unwired: 1 out]
        }
      }
    }
    frame #8 {
      n111 = local read "AutoMode"() -> (w275:string)
      n112 = case shown="\"LeftScale\"" w275 {
        frame "LeftSwitch" {
          n113 = call "Release.vi"("Release"=0.0) -> ()  [unwired: 11 in]
          n114 = Wait (ms)(milliseconds to wait=u32 1000) -> ()  [unwired: 1 out]
        }
        frame "LeftScale" {
          n115 = disable-structure shown="Disabled" {
            frame Disabled {
              n116 = call "GripperActuator.vi"(8:1.0 ("Actuator")) -> ()  [unwired: 11 in]
            }
            frame Enabled {
            }
          }
          n117 = Wait (ms)(milliseconds to wait=u32 1000) -> ()  [unwired: 1 out]
        }
        frame "Baseline", Default {
          n118 = Wait (ms)(milliseconds to wait=u32 1000) -> ()  [unwired: 1 out]
        }
        frame "RightScale" {
          n119 = disable-structure shown="Disabled" {
            frame Disabled {
              n120 = call "GripperActuator.vi"(8:1.0 ("Actuator")) -> ()  [unwired: 11 in]
            }
            frame Enabled {
            }
          }
          n121 = Wait (ms)(milliseconds to wait=u32 1000) -> ()  [unwired: 1 out]
        }
        frame "RightSwitch" {
          n122 = call "Release.vi"("Release"=0.0) -> ()  [unwired: 11 in]
          n123 = Wait (ms)(milliseconds to wait=u32 1000) -> ()  [unwired: 1 out]
        }
      }
      n124 = call "Slide Prevention.vi"("Slide?"=TRUE) -> ()  [unwired: 11 in]
    }
  }
